vi "Node.vi"(8 "error in (no error)":errorcluster, 11 "Group in":refnum<class "Group.lvclass">) -> (0 "error out":errorcluster, 2 "Node":string, 3 "Group out":refnum<class "Group.lvclass">)   [LabVIEW 2020, in "Vecto.lvlib" / "Group.lvclass"]
uses:
  Group.lvclass
  Group Config/Group Config.lvclass
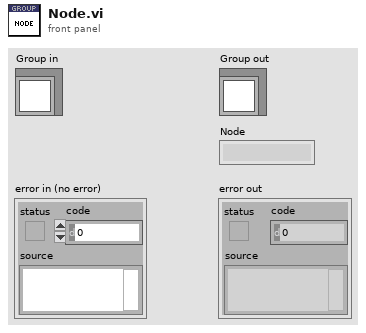
[diagram p1: front panel]
types:
  T1 = typedef "VectoConfig.lvlib/Group Info.ctl" = cluster{"System":string, "Cluster":string, "Node":string, "Task":string, "Name":string}
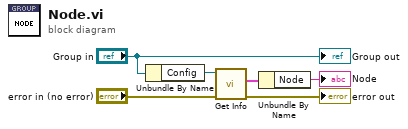
[diagram p0: block diagram]
diagram:
  n1 = Unbundle By Name("Group in") -> ("Config"=w5:refnum<class "Group Config.lvclass">)
  n2 = call "Get Info.vi"("error in (no error)"="error in (no error)", "Group Config in"=w5) -> ("error out"=→"error out":errorcluster, "Info"=w4:T1)  [unwired: 7 in, 1 out]
  n3 = Unbundle By Name(w4) -> ("Node"=→"Node":string)
  "Group out" <- "Group in"
